vi "Read Scalar Data.vi"(8 "error in (no error)":errorcluster, 9 "Values":dbl[](array[numeric]), 10 "session in":u32, 11 "Cluster":T1 {"Data Type" format="%.0x"}) -> (0 "error out":errorcluster, 1 "Values":dbl[](array[numeric]), 2 "session out":u32, 3 "Cluster":T1 {"Data Type" format="%.0x"})   [LabVIEW 2018, in "FPGA Addon Engine.lvlib"]
uses:
  FPGA Addon Engine.lvlib
  Types/Register Settings.ctl
  Addon Shared/Types/Data Type.ctl
  Addon Shared/Types/Scalar Type.ctl
  APIs/FPGA Register IO/Read Methods/Read Data Register/Instances/Read I8.vi
  APIs/FPGA Register IO/Read Methods/Read Data Register/Instances/Read I16.vi
  APIs/FPGA Register IO/Read Methods/Read Data Register/Instances/Read I32.vi
  APIs/FPGA Register IO/Read Methods/Read Data Register/Instances/Read I64.vi
  APIs/FPGA Register IO/Read Methods/Read Data Register/Instances/Read U8.vi
  APIs/FPGA Register IO/Read Methods/Read Data Register/Instances/Read U16.vi
  APIs/FPGA Register IO/Read Methods/Read Data Register/Instances/Read U32.vi
  APIs/FPGA Register IO/Read Methods/Read Data Register/Instances/Read U64.vi
  APIs/FPGA Register IO/Read Methods/Read Data Register/Instances/Read SGL.vi
  APIs/FPGA Register IO/Read Methods/Read Data Register/Instances/Read Boolean.vi
  <vilib>/Utility/error.llb/Error Cluster From Error Code.vi
  <vilib>/rvi/errors/niLvFpgaAdjustHostInterfaceError.vi
  <vilib>/rvi/interface/nirviReadWriteControl/nirviReadWriteControl.xnode
  NiFpgaLv.dll
  <vilib>/rvi/interface/Simulation/niFpgaSimulationCallBeginRW.vi
  APIs/FPGA Register IO/FPGA Register IO.lvlib
  Addon Shared/FPGA Addon Shared.lvlib
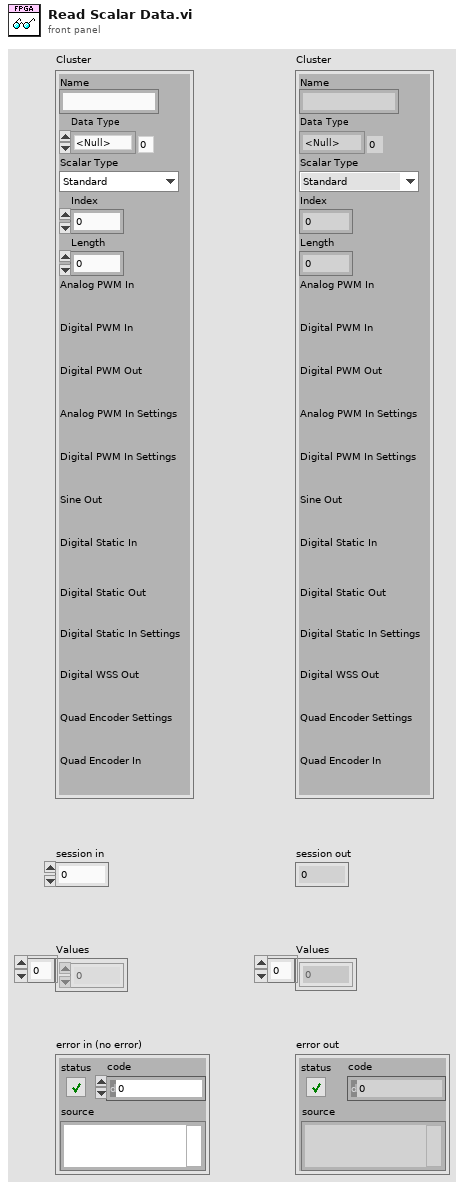
[diagram p1: front panel]
types:
  T1 = typedef "FPGA Addon Engine.lvlib/Register Settings.ctl" = cluster{"Name":string, "Data Type":T2, "Scalar Type":T3, "Index":i32, "Length":i32, "Analog PWM In":refnum<k20>, "Digital PWM In":refnum<k20>, "Digital PWM Out":refnum<k20>, "Analog PWM In Settings":refnum<k20>, "Digital PWM In Settings":refnum<k20>, "Sine Out":refnum<k20>, "Digital Static In":refnum<k20>, "Digital Static Out":refnum<k20>, "Digital Static In Settings":refnum<k20>, "Digital WSS Out":refnum<k20>, "Quad Encoder Settings":refnum<k20>, "Quad Encoder In":refnum<k20>}
  T2 = typedef "FPGA Addon Shared.lvlib/Data Type.ctl" = enum8{"<Null>", "I8", "I16", "I32", "I64", "U8", "U16", "U32", "U64", "SGL", "Boolean", "Analog PWM In Settings", "Analog PWM In", "Digital PWM In Settings", "Digital PWM In", "Digital PWM Out", "Sine Out", "FXP+/-24.5", "FXP+/-16.5", "FXP+/-32.8", "FXP+/-64.32", "FXP+/-16.7", "FXP+/-20.5", "FXP+/-27.5", "FXP+/-32.16", "FXP+16.3", "FXP+18.3", "Digital Static In", "Digital Static Out", "Digital Static In Settings", "Digital WSS Out", "Quad Encoder Settings", "Quad Encoder In", "Group"}
  T3 = typedef "FPGA Addon Shared.lvlib/Scalar Type.ctl" = enum16{"Standard", "Bitpacked"}
  T4 = cluster{"ACTIVE TICKS":u32, "INACTIVE TICKS":u32, "ACQ TICKS":u32, "ACTIVE VOLTAGE":fxp<+/-,32,8>, "INACTIVE VOLTAGE":fxp<+/-,32,8>}
  T5 = cluster{"ACTIVE TICKS":u32, "INACTIVE TICKS":u32, "ACQ TICKS":u32}
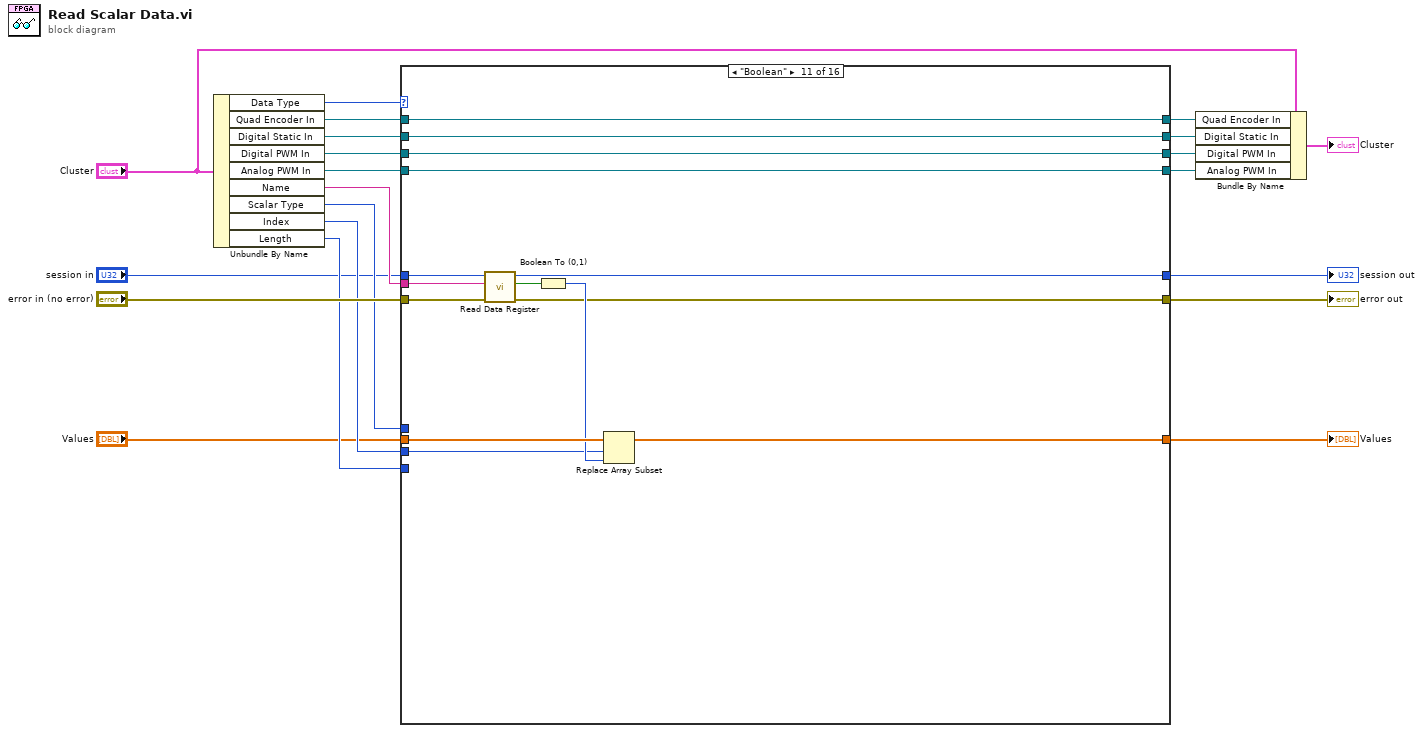
[diagram p0: block diagram]
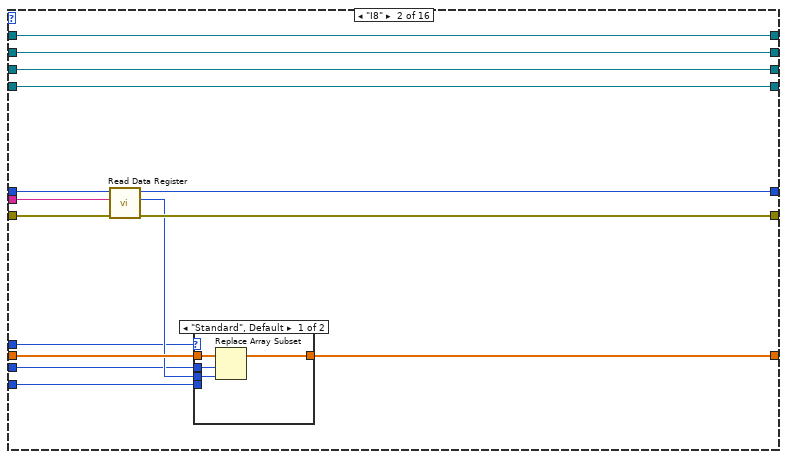
[diagram p3: hidden frame]
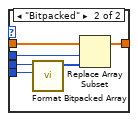
[diagram p4: hidden frame]
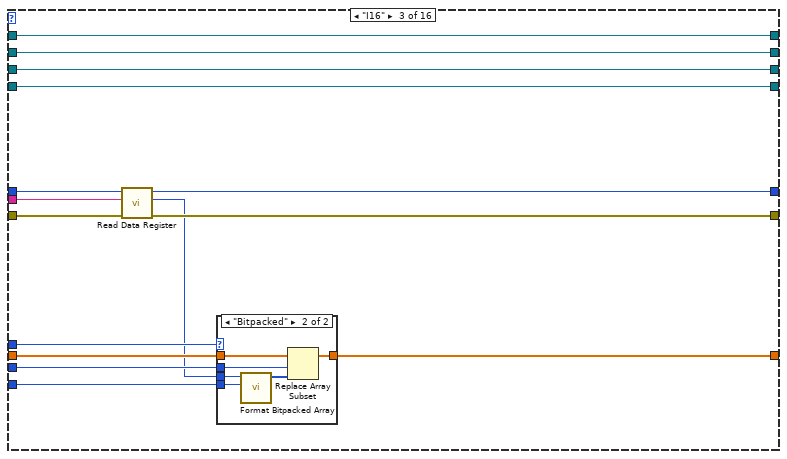
[diagram p5: hidden frame]
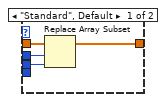
[diagram p6: hidden frame]
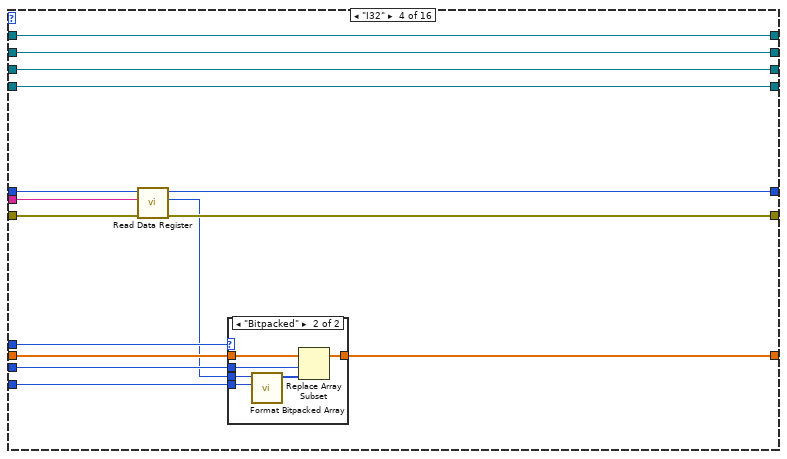
[diagram p7: hidden frame]
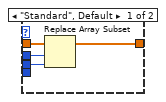
[diagram p8: hidden frame]
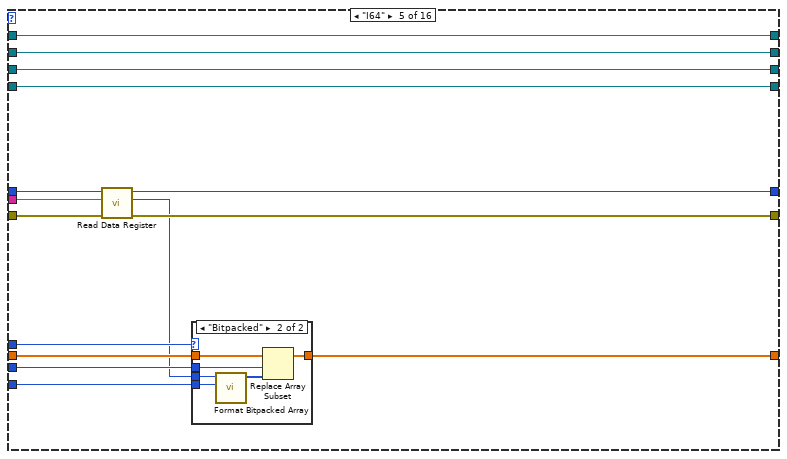
[diagram p9: hidden frame]
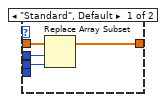
[diagram p10: hidden frame]
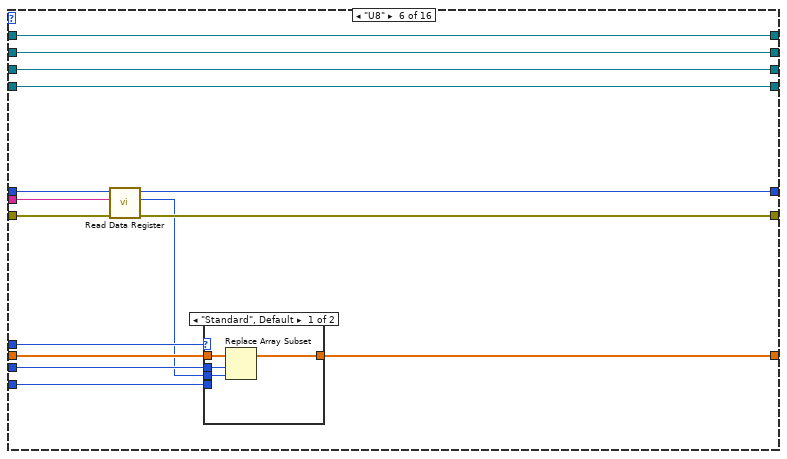
[diagram p11: hidden frame]
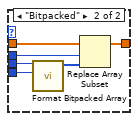
[diagram p12: hidden frame]
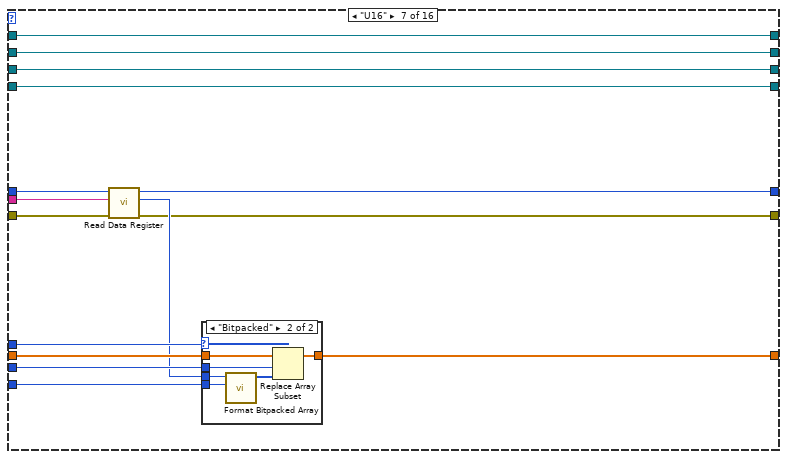
[diagram p13: hidden frame]
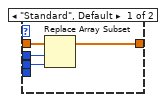
[diagram p14: hidden frame]
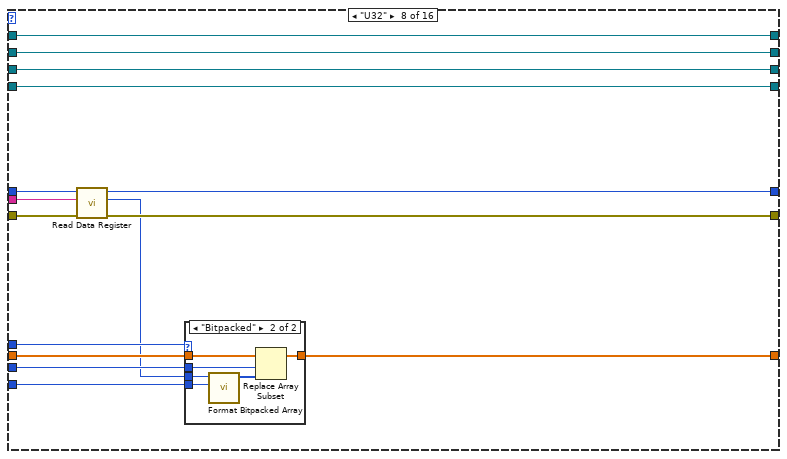
[diagram p15: hidden frame]
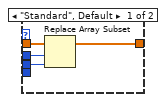
[diagram p16: hidden frame]
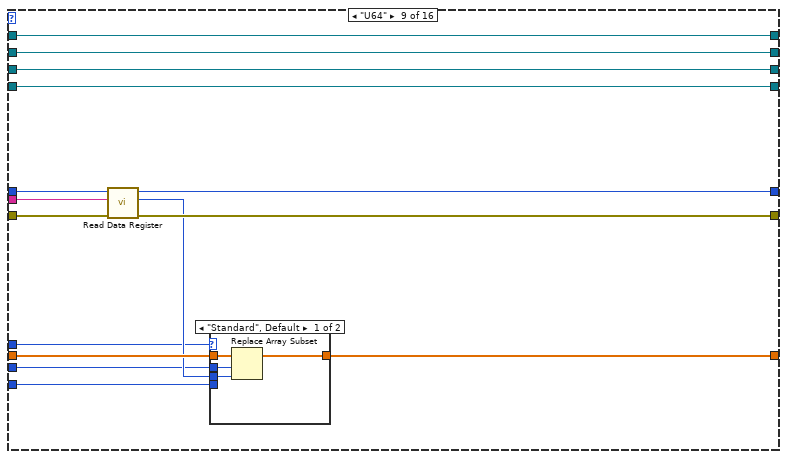
[diagram p17: hidden frame]
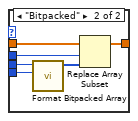
[diagram p18: hidden frame]
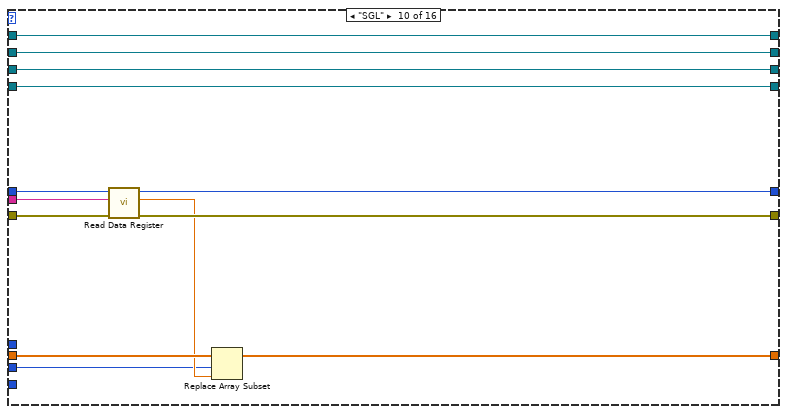
[diagram p19: hidden frame]
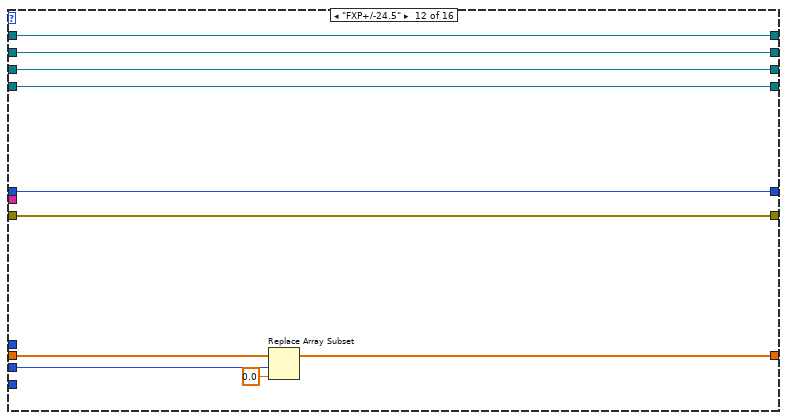
[diagram p20: hidden frame]
diagram:
  n1 = Unbundle By Name("Cluster") -> ("Data Type"=w6:T2, "Quad Encoder In"=w5:refnum<k20>, "Digital Static In"=w8:refnum<k20>, "Digital PWM In"=w10:refnum<k20>, "Analog PWM In"=w11:refnum<k20>, "Name"=w3:string, "Scalar Type"=w15:T3, "Index"=w16:i32, "Length"=w17:i32)
  n2 = case shown="\"Boolean\"" w6 {
    tunnel: "error in (no error)" -> [w28 w36 w61 w84 w109 w134 w159 w186 w211 w235 w248 w265 w279 w311 w348 w366]
    tunnel: [w28 w34 w60 w83 w108 w133 w156 w185 w210 w234 w247 w265 w278 w310 w347 w365] -> w20
    tunnel: w17 -> [_ w42 w67 w91 w117 w142 w168 w191 w218 _ _ _ _ _ _ _]
    tunnel: w16 -> [_ w31 w57 w85 w110 w135 w160 w182 w206 w232 w244 w257 w266 w280 w318 w354]
    tunnel: w15 -> [_ w32 w58 w86 w111 w136 w161 w183 w207 _ _ _ _ _ _ _]
    tunnel: "Values" -> [w27 w43 w68 w93 w118 w143 w167 w193 w217 w241 w255 w264 w277 w295 w332 w363]
    tunnel: [w27 w41 w66 w92 w116 w141 w166 w192 w216 w240 w253 w263 w276 w294 w331 w362] -> w13
    tunnel: [w26 w39 w64 w89 w114 w139 w164 w189 w214 w238 w251 w261 w274 w308 w329 w361] -> w12
    tunnel: w11 -> [w26 w39 w64 w89 w114 w139 w164 w189 w214 w238 w251 w261 w274 w309 w329 w361]
    tunnel: w10 -> [w25 w40 w65 w90 w115 w140 w165 w190 w215 w239 w252 w262 w275 w312 w328 w359]
    tunnel: [w25 w40 w65 w90 w115 w140 w165 w190 w215 w239 w252 w262 w275 w312 w327 w359] -> w9
    tunnel: w8 -> [w24 w38 w63 w88 w113 w138 w163 w188 w213 w237 w250 w260 w272 w283 w321 w360]
    tunnel: [w24 w38 w63 w88 w113 w138 w163 w188 w213 w237 w250 w260 w270 w283 w321 w360] -> w7
    tunnel: w5 -> [w23 w37 w62 w87 w112 w137 w162 w187 w212 w236 w249 w259 w268 w282 w320 w358]
    tunnel: [w23 w37 w62 w87 w112 w137 w162 w187 w212 w236 w249 w259 w268 w282 w320 w357] -> w4
    tunnel: w3 -> [_ w35 w59 w81 w106 w131 w158 w184 w208 w231 w245 _ _ _ _ _]
    tunnel: "session in" -> [w22 w30 w55 w80 w105 w130 w155 w180 w205 w230 w243 w258 w267 w281 w319 w355]
    tunnel: [w22 w29 w54 w79 w104 w129 w154 w179 w204 w229 w242 w258 w267 w281 w319 w355] -> w1
    frame "<Null>", Default {
    }
    frame "I8" {
      n3 = call-poly "Read Data Register.vi"("error in"=w36, "register name"=w35, "session in"=w30) -> ("error out"=w34:errorcluster, "value out"=w33:i8, "session out"=w29:u32)  [unwired: 6 in]
      n4 = case shown="\"Standard\", Default" w32 {
        tunnel: w43 -> [w47 w52]
        tunnel: [w46 w51] -> w41
        tunnel: w42 -> [_ w53]
        tunnel: w33 -> [w44 w49]
        tunnel: w31 -> [w45 w48]
        frame "Standard", Default {
          n5 = Replace Array Subset(array=w47, new element=w44, index=w45) -> (w46:dbl[])
        }
        frame "Bitpacked" {
          n6 = call "Format Bitpacked Array.vi"("Length"=w53, "Value"=w49) -> ("Array"=w50:i16[])  [unwired: 9 in]
          n7 = Replace Array Subset(array=w52, new element=w50, index=w48) -> (w51:dbl[])
        }
      }
    }
    frame "I16" {
      n8 = call-poly "Read Data Register.vi"("error in"=w61, "register name"=w59, "session in"=w55) -> ("error out"=w60:errorcluster, "value out"=w56:i16, "session out"=w54:u32)  [unwired: 6 in]
      n9 = case shown="\"Bitpacked\"" w58 {
        tunnel: w68 -> [w72 w77]
        tunnel: [w71 w76] -> w66
        tunnel: w56 -> [w70 w73]
        tunnel: w57 -> [w69 w74]
        tunnel: w67 -> [_ w78]
        frame "Standard", Default {
          n10 = Replace Array Subset(array=w72, new element=w70, index=w69) -> (w71:dbl[])
        }
        frame "Bitpacked" {
          n11 = call "Format Bitpacked Array.vi"("Length"=w78, "Value"=w73) -> ("Array"=w75:i16[])  [unwired: 9 in]
          n12 = Replace Array Subset(array=w77, new element=w75, index=w74) -> (w76:dbl[])
        }
      }
    }
    frame "I32" {
      n13 = call-poly "Read Data Register.vi"("error in"=w84, "register name"=w81, "session in"=w80) -> ("error out"=w83:errorcluster, "value out"=w82:i32, "session out"=w79:u32)  [unwired: 6 in]
      n14 = case shown="\"Bitpacked\"" w86 {
        tunnel: w93 -> [w97 w101]
        tunnel: [w96 w100] -> w92
        tunnel: w82 -> [w95 w103]
        tunnel: w85 -> [w94 w98]
        tunnel: w91 -> [_ w102]
        frame "Standard", Default {
          n15 = Replace Array Subset(array=w97, new element=w95, index=w94) -> (w96:dbl[])
        }
        frame "Bitpacked" {
          n16 = call "Format Bitpacked Array.vi"("Length"=w102, "Value"=w103) -> ("Array"=w99:i16[])  [unwired: 9 in]
          n17 = Replace Array Subset(array=w101, new element=w99, index=w98) -> (w100:dbl[])
        }
      }
    }
    frame "I64" {
      n18 = call-poly "Read Data Register.vi"("error in"=w109, "register name"=w106, "session in"=w105) -> ("error out"=w108:errorcluster, "value out"=w107:i64, "session out"=w104:u32)  [unwired: 6 in]
      n19 = case shown="\"Bitpacked\"" w111 {
        tunnel: w118 -> [w122 w126]
        tunnel: [w121 w125] -> w116
        tunnel: w107 -> [w120 w128]
        tunnel: w110 -> [w119 w123]
        tunnel: w117 -> [_ w127]
        frame "Standard", Default {
          n20 = Replace Array Subset(array=w122, new element=w120, index=w119) -> (w121:dbl[])
        }
        frame "Bitpacked" {
          n21 = call "Format Bitpacked Array.vi"("Length"=w127, "Value"=w128) -> ("Array"=w124:i16[])  [unwired: 9 in]
          n22 = Replace Array Subset(array=w126, new element=w124, index=w123) -> (w125:dbl[])
        }
      }
    }
    frame "U8" {
      n23 = call-poly "Read Data Register.vi"("error in"=w134, "register name"=w131, "session in"=w130) -> ("error out"=w133:errorcluster, "value out"=w132:u8, "session out"=w129:u32)  [unwired: 6 in]
      n24 = case shown="\"Standard\", Default" w136 {
        tunnel: w143 -> [w147 w152]
        tunnel: [w146 w151] -> w141
        tunnel: w142 -> [_ w153]
        tunnel: w135 -> [w145 w149]
        tunnel: w132 -> [w144 w148]
        frame "Standard", Default {
          n25 = Replace Array Subset(array=w147, new element=w144, index=w145) -> (w146:dbl[])
        }
        frame "Bitpacked" {
          n26 = call "Format Bitpacked Array.vi"("Length"=w153, "Value"=w148) -> ("Array"=w150:i16[])  [unwired: 9 in]
          n27 = Replace Array Subset(array=w152, new element=w150, index=w149) -> (w151:dbl[])
        }
      }
    }
    frame "U16" {
      n28 = call-poly "Read Data Register.vi"("error in"=w159, "register name"=w158, "session in"=w155) -> ("error out"=w156:errorcluster, "value out"=w157:u16, "session out"=w154:u32)  [unwired: 6 in]
      n29 = case shown="\"Bitpacked\"" w161 {
        tunnel: w167 -> [w172 w176]
        tunnel: [w171 w175] -> w166
        tunnel: w157 -> [w170 w178]
        tunnel: w160 -> [w169 w173]
        tunnel: w168 -> [_ w177]
        frame "Standard", Default {
          n30 = Replace Array Subset(array=w172, new element=w170, index=w169) -> (w171:dbl[])
        }
        frame "Bitpacked" {
          n31 = call "Format Bitpacked Array.vi"("Length"=w177, "Value"=w178) -> ("Array"=w174:i16[])  [unwired: 9 in]
          n32 = Replace Array Subset(array=w176, new element=w174, index=w173) -> (w175:dbl[])
        }
      }
    }
    frame "U32" {
      n33 = call-poly "Read Data Register.vi"("error in"=w186, "register name"=w184, "session in"=w180) -> ("error out"=w185:errorcluster, "value out"=w181:u32, "session out"=w179:u32)  [unwired: 6 in]
      n34 = case shown="\"Bitpacked\"" w183 {
        tunnel: w193 -> [w197 w201]
        tunnel: [w196 w200] -> w192
        tunnel: w181 -> [w195 w203]
        tunnel: w182 -> [w194 w198]
        tunnel: w191 -> [_ w202]
        frame "Standard", Default {
          n35 = Replace Array Subset(array=w197, new element=w195, index=w194) -> (w196:dbl[])
        }
        frame "Bitpacked" {
          n36 = call "Format Bitpacked Array.vi"("Length"=w202, "Value"=w203) -> ("Array"=w199:i16[])  [unwired: 9 in]
          n37 = Replace Array Subset(array=w201, new element=w199, index=w198) -> (w200:dbl[])
        }
      }
    }
    frame "U64" {
      n38 = call-poly "Read Data Register.vi"("error in"=w211, "register name"=w208, "session in"=w205) -> ("error out"=w210:errorcluster, "value out"=w209:u64, "session out"=w204:u32)  [unwired: 6 in]
      n39 = case shown="\"Standard\", Default" w207 {
        tunnel: w217 -> [w222 w226]
        tunnel: [w221 w225] -> w216
        tunnel: w209 -> [w220 w228]
        tunnel: w206 -> [w219 w223]
        tunnel: w218 -> [_ w227]
        frame "Standard", Default {
          n40 = Replace Array Subset(array=w222, new element=w220, index=w219) -> (w221:dbl[])
        }
        frame "Bitpacked" {
          n41 = call "Format Bitpacked Array.vi"("Length"=w227, "Value"=w228) -> ("Array"=w224:i16[])  [unwired: 9 in]
          n42 = Replace Array Subset(array=w226, new element=w224, index=w223) -> (w225:dbl[])
        }
      }
    }
    frame "SGL" {
      n43 = call-poly "Read Data Register.vi"("error in"=w235, "register name"=w231, "session in"=w230) -> ("error out"=w234:errorcluster, "value out"=w233:sgl, "session out"=w229:u32)  [unwired: 6 in]
      n44 = Replace Array Subset(array=w241, new element=w233, index=w232) -> (w240:dbl[])
    }
    frame "Boolean" {
      n45 = call-poly "Read Data Register.vi"("error in"=w248, "register name"=w245, "session in"=w243) -> ("error out"=w247:errorcluster, "value out"=w246:bool, "session out"=w242:u32)  [unwired: 6 in]
      n46 = Boolean To (0,1)(Boolean=w246) -> (0, 1=w254:i16)
      n47 = Replace Array Subset(array=w255, new element=w254, index=w244) -> (w253:dbl[])
    }
    frame "FXP+/-24.5" {
      n48 = Replace Array Subset(array=w264, new element=0.0 ("new element/subarray"), index=w257) -> (w263:dbl[])
    }
    frame "Digital Static In" {
      n49 = xnode "Read/Write Control"("FPGA VI Reference In"=w272, "error in"=w279) -> ("FPGA VI Reference Out"=w270:refnum<k20>, "error out"=w278:errorcluster, "Value"=w273:cluster{"STATE":bool})
      n50 = Unbundle By Name(w273) -> ("STATE"=w271:bool)
      n51 = Boolean To (0,1)(Boolean=w271) -> (0, 1=w269:i16)
      n52 = Replace Array Subset(array=w277, new element=w269, index=w266) -> (w276:dbl[])
    }
    frame "Analog PWM In" {
      w302 = 2.5000000292152436e-08 ("y")
      n53 = xnode "Read/Write Control"("FPGA VI Reference In"=w309, "error in"=w311) -> ("FPGA VI Reference Out"=w308:refnum<k20>, "error out"=w310:errorcluster, "Value"=w291:T4)
      n54 = Unbundle By Name(w291) -> ("ACTIVE TICKS"=w290:u32, "INACTIVE TICKS"=w289:u32, "ACQ TICKS"=w288:u32, "ACTIVE VOLTAGE"=w287:fxp<+/-,32,8>, "INACTIVE VOLTAGE"=w286:fxp<+/-,32,8>)
      n55 = Add(x=w290, y=w289) -> (x+y=w304:u32)
      n56 = Compound Arithmetic op=MULTIPLY(w304, w288, w302) -> (w305:dbl)
      n57 = Divide(x=w290, y=w304) -> (x/y=w298:dbl)
      n58 = Compound Arithmetic op=MULTIPLY(w290, w288, w302) -> (w303:dbl)
      n59 = Multiply(x=100.0, y=w298) -> (x*y=w297:dbl)
      n60 = Equal?(x=0.0, y=w305) -> (x = y?=w301:bool)
      n61 = Reciprocal(x=w305) -> (1/x=w306:dbl)
      n62 = case shown="False" w301 {
        tunnel: [w313 w317] -> w285
        tunnel: [w314 w317] -> w292
        tunnel: [w316 w317] -> w284
        tunnel: w305 -> [w316 _]
        tunnel: [w315 w317] -> w296
        tunnel: w303 -> [w315 _]
        tunnel: w297 -> [w314 _]
        tunnel: w306 -> [w313 _]
        tunnel: 0.0 ("x") -> [_ w317]
        frame False {
        }
        frame True {
        }
      }
      n63 = Build Array(w285, w284, w292, w296, w287, w286) -> (w293:dbl[])
      n64 = Replace Array Subset(array=w295, new element=w293, index=w280) -> (w294:dbl[])
    }
    frame "Digital PWM In" {
      w341 = 2.5000000292152436e-08 ("y")
      n65 = xnode "Read/Write Control"("FPGA VI Reference In"=w328, "error in"=w348) -> ("FPGA VI Reference Out"=w327:refnum<k20>, "error out"=w347:errorcluster, "Value"=w334:T5)
      n66 = Unbundle By Name(w334) -> ("ACTIVE TICKS"=w325:u32, "INACTIVE TICKS"=w324:u32, "ACQ TICKS"=w337:u32)
      n67 = Add(x=w325, y=w324) -> (x+y=w343:u32)
      n68 = Compound Arithmetic op=MULTIPLY(w343, w337, w341) -> (w344:dbl)
      n69 = Divide(x=w325, y=w343) -> (x/y=w336:dbl)
      n70 = Compound Arithmetic op=MULTIPLY(w325, w337, w341) -> (w342:dbl)
      n71 = Multiply(x=100.0, y=w336) -> (x*y=w335:dbl)
      n72 = Equal?(x=0.0, y=w344) -> (x = y?=w340:bool)
      n73 = Reciprocal(x=w344) -> (1/x=w345:dbl)
      n74 = case shown="False" w340 {
        tunnel: [w349 w353] -> w323
        tunnel: [w350 w353] -> w326
        tunnel: [w352 w353] -> w322
        tunnel: w344 -> [w352 _]
        tunnel: [w351 w353] -> w333
        tunnel: w342 -> [w351 _]
        tunnel: w335 -> [w350 _]
        tunnel: w345 -> [w349 _]
        tunnel: 0.0 ("x") -> [_ w353]
        frame False {
        }
        frame True {
        }
      }
      n75 = Build Array(w323, w322, w326, w333) -> (w330:dbl[])
      n76 = Replace Array Subset(array=w332, new element=w330, index=w318) -> (w331:dbl[])
    }
    frame "Quad Encoder In" {
      n77 = xnode "Read/Write Control"("FPGA VI Reference In"=w358, "error in"=w366) -> ("FPGA VI Reference Out"=w357:refnum<k20>, "error out"=w365:errorcluster, "Value"=w364:cluster{"POSITION":i32})
      n78 = Unbundle By Name(w364) -> ("POSITION"=w356:i32)
      n79 = Replace Array Subset(array=w363, new element=w356, index=w354) -> (w362:dbl[])
    }
  }
  "error out" <- w20
  "Values" <- w13
  "session out" <- w1
  n80 = Bundle By Name(cluster="Cluster", "Quad Encoder In"=w4, "Digital Static In"=w7, "Digital PWM In"=w9, "Analog PWM In"=w12) -> (→"Cluster":T1)
